vi "Array of Variants to Cluster Variant.vi"(8 "error in (no error)":errorcluster, 11 "[Variant]":variant[](array[variant])) -> (0 "error out":errorcluster, 3 "Cluster Variant":variant)   [LabVIEW 2018, in "TwinCAT ADS.lvclass"]
uses:
  TwinCAT ADS.lvclass
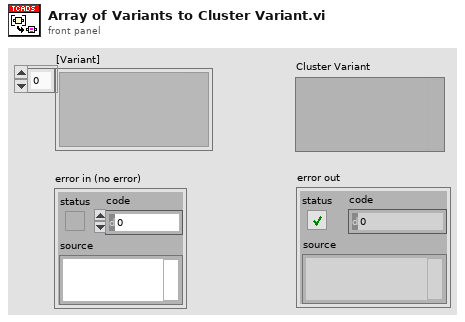
[diagram p1: front panel]
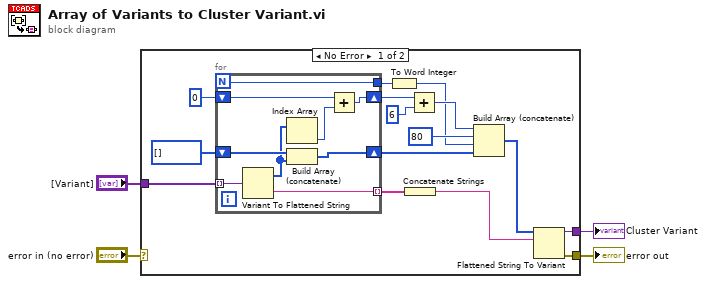
[diagram p0: block diagram]
diagram:
  n1 = case shown="No Error" "error in (no error)" {
    selector: "error in (no error)" -> [_ w29]
    tunnel: [w9 w29] -> w4
    tunnel: [w8 _] -> w3
    tunnel: "[Variant]" -> [w7 _]
    frame No Error {
      n2 = for {
        N -> [w27]
        tunnel: w7 -> [w28] mode=indexing
        shift-right: [w20] -> w11
        shift-left: i16[] [] ("type string") -> [w26]
        tunnel: [w27] -> w13
        shift-right: [w22] -> w17
        shift-left: i16 0 -> [w23]
        tunnel: [w21] -> w6 mode=indexing
        n3 = Variant To Flattened String(Variant=w28) -> (data string=w21:string, 1:w25:i16[])
        n4 = Index Array(array=w25) -> (element=w24:i16)  [unwired: 1 in]
        n5 = Build Array (concatenate)(w26, w25) -> (w20:i16[])
        n6 = Add(x=w23, y=w24) -> (x+y=w22:i16)
      }
      n7 = To Word Integer(number=w13) -> (16bit integer=w12:i16)
      n8 = Concatenate Strings(w6) -> (w5:string)
      n9 = Add(x=w17, y=i16 6) -> (x+y=w15:i16)
      n10 = Build Array (concatenate)(w15, i16 80, w12, w11) -> (w10:i16[])
      n11 = Flattened String To Variant(6:w5, 7:w10) -> (0:w9:errorcluster, 3:w8:variant)  [unwired: 1 in]
    }
    frame Error {
    }
  }
  "Cluster Variant" <- w3
  "error out" <- w4
